vi "FTW-JSON-ObjectManip-AddPair.vi"(0 "Input JSON Object":string, 5 "Key":string, 7 "Value":string, 11 "error in":errorcluster) -> (4 "Output JSON Object":string, 15 "error out":errorcluster)   [LabVIEW 2013]
uses:
  FTW-JSON.lvclass
panel:
  # "Inputs"
  # "Outputs"
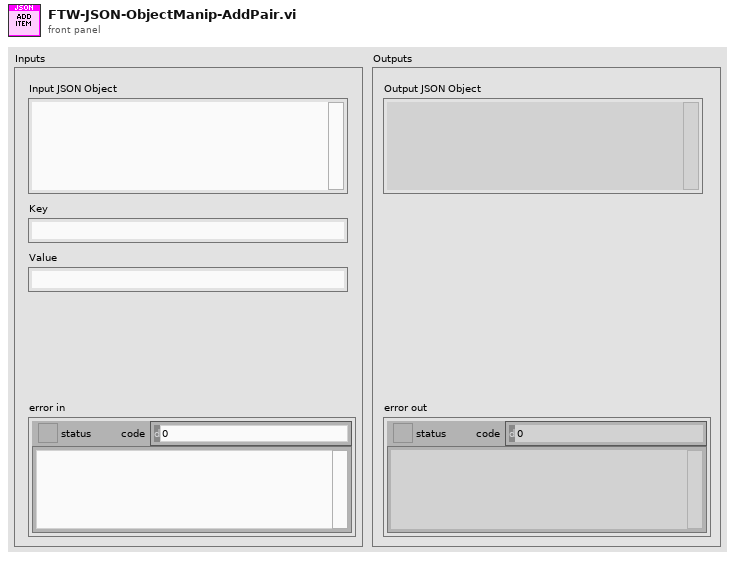
[diagram p1: front panel]
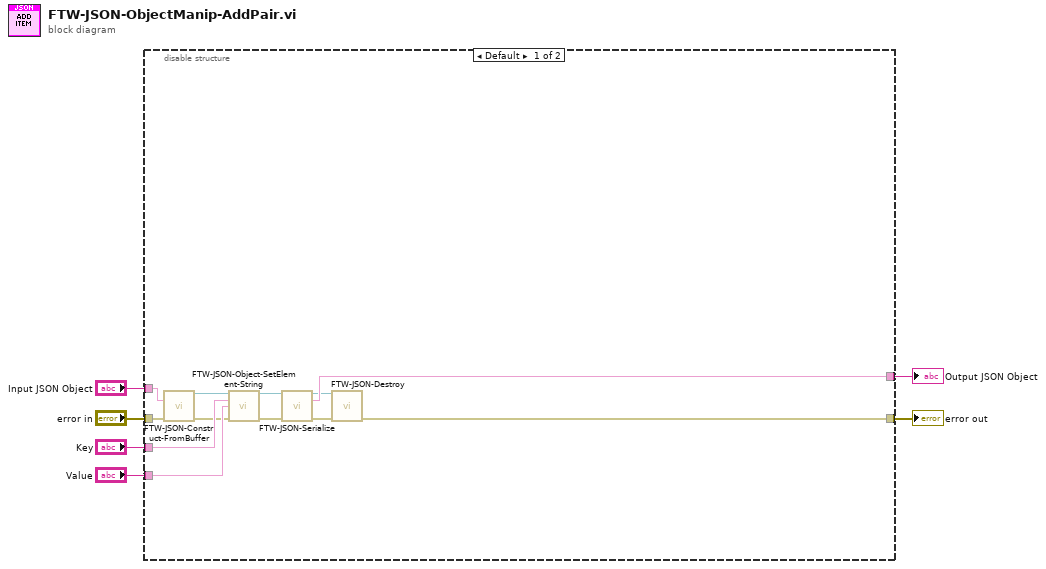
[diagram p0: block diagram]
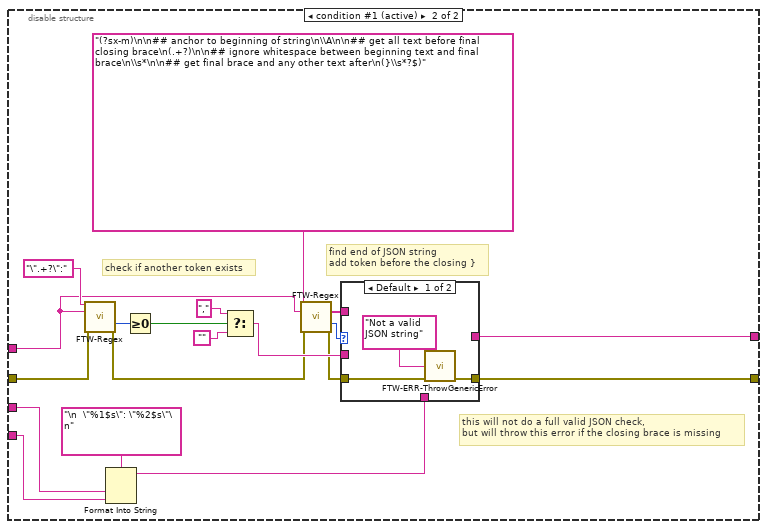
[diagram p2: hidden frame]
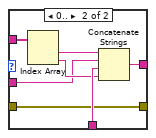
[diagram p3: hidden frame]
diagram:
  n1 = disable-structure shown="Default" {
    disable-tunnel: "Key" -> [w18 w29]
    disable-tunnel: "Value" -> [w17 w28]
    disable-tunnel: "Input JSON Object" -> [w16 w20]
    disable-tunnel: "error in" -> [w15 w27]
    disable-tunnel: [w14 w30] -> w2
    disable-tunnel: [w13 w31] -> w1
    frame condition #0 {
      n2 = call "FTW-JSON-Construct-FromBuffer.vi"("JSON String (UTF-8)"=w16, "error in"=w15) -> ("JSON Object"=w10:refnum<class "FTW-JSON.lvclass">, "error out"=w8:errorcluster)  [unwired: 12 in]
      n3 = call "FTW-JSON-Object-SetElement-String.vi"("JSON Object"=w10, "Key"=w18, "Value"=w17, "error in"=w8) -> ("JSON Object out"=w9:refnum<class "FTW-JSON.lvclass">, "error out"=w7:errorcluster)  [unwired: 10 in]
      n4 = call "FTW-JSON-Serialize.vi"("JSON Object"=w9, "error in"=w7) -> ("JSON Object out"=w12:refnum<class "FTW-JSON.lvclass">, "JSON String (UTF-8)"=w13:string, "error out"=w11:errorcluster)  [unwired: 11 in]
      n5 = call "FTW-JSON-Destroy.vi"("JSON Object"=w12, "error in"=w11) -> ("error out"=w14:errorcluster)  [unwired: 13 in]
    }
    frame condition #1 (active) {
      # "this will not do a full valid JSON check,\nbut will throw this error if the closing brace is missing"
      # "find end of JSON string\nadd token before the closing }"
      # "check if another token exists"
      n6 = call "FTW-Regex.vi"("Regular Expression"="\".+?\":" ("format string"), "Input String"=w20, "error in"=w27) -> ("Offset after Match"=w19:i32, "error out"=w25:errorcluster)  [unwired: 8 in, 3 out]
      n7 = Format Into String(format string="\n  \"%1$s\": \"%2$s\"\n", w29, w28) -> (resulting string=w36:string)  [unwired: 2 in, 1 out]
      n8 = Greater Or Equal To 0?(x=w19) -> (x >= 0?=w33:bool)
      n9 = Select(t="," ("format string"), s=w33, f="") -> (s? t:f=w37:string)
      n10 = call "FTW-Regex.vi"("Regular Expression"="(?sx-m)\n\n## anchor to beginning of string\n\\A\n\n## get all text before final closing brace\n(.+?)\n\n## ignore whitespace between beginning text and final brace\n\\s*\n\n## get final brace and any other text after\n(}\\s*?$)" ("format string"), "Input String"=w20, "error in"=w25) -> ("Submatches"=w22:string[], "Offset after Match"=w21:i32, "error out"=w24:errorcluster)  [unwired: 8 in, 2 out]
      n11 = case shown="Default" w21 {
        tunnel: w22 -> [_ w47]
        tunnel: w36 -> [_ w45]
        tunnel: [_ w43] -> w31
        tunnel: w24 -> [w40 w42]
        tunnel: w37 -> [_ w41]
        tunnel: [w39 w42] -> w30
        frame Default {
          n12 = call "FTW-ERR-ThrowGenericError.vi"("Error Message"="Not a valid JSON string", "error in"=w40) -> ("error out"=w39:errorcluster)  [unwired: 13 in]
        }
        frame 0.. {
          n13 = Index Array(array=w47) -> (element #1=w46:string, element #2=w44:string)  [unwired: 2 in]
          n14 = Concatenate Strings(w46, w41, w45, w44) -> (w43:string)
        }
      }
    }
  }
  "error out" <- w2
  "Output JSON Object" <- w1
